vi "Controller Data Server Loop.vi"(4 "Log File Reference":refnum<file>, 7 "Sync Objects":T1, 8 "error in (no error)":errorcluster, 11 "FOFB Configuration":T5={"FOFB Parameters"={"Network"={"FOFB Controller IP"="", "LNLS Control Network IP"="", "LNLS Control Network Power Supplies TCP Port"=0, "LNLS Control Network FOFB Configuration TCP Port"=0, "Data Server TCP Port"=0, "Monitoring Data TCP Port"=0, "Configuration GUI TCP Port"=0, "TCP Listening Timeout"=0}, "Fast Acquisition"={"Acquisition Period"=0, "Data Buffer Size"=0, "Monitoring Period"=0}, "Response Matrix Measurement"={"Step Amplitude"=0.0, "Time Between Steps"=0, "Step Duration"=0, "Number of Averages"=0}, "Correction Algorithm"={"Correction Period"=0, "Reference Orbit Path"=path "", "Response Matrix Path"=path "", "Correction Matrix Path"=path "", "Horizontal Correction Factor"=0.0, "Vertical Correction Factor"=0.0, "Beam Current FOFB Threshold"=0.0, "Decouple H-V"=FALSE, "Use Additional BPM LPF"=FALSE, "BPM LPF Cutoff"=0.0}, "Acquisition Network"=[], "Actuation Network"=[]}, "Number of Acquisition Chassis"=0, "Number of Actuation Chassis"=0, "Number of BPM Readings"=0, "BPM Reading Names"=[], "Selected BPM Readings"=[0, 1, 2, 3, 4, 5, 6, 7, 8, 9, 10, 11, 12, 13, 14, 15, 16, 17, 18, 19, 20, 21, 22, 23, 24, 25, 26, 27, 28, 29, 30, 31, 32, 33, 34, 35, 36, 37, 38, 39, 40, 41, 42, 43, 44, 45, 46, 47, 48, 49], "Number of Correctors"=0, "Corrector Names"=[], "Selected Correctors"=[0, 1, 2, 3, 4, 5, 6, 7, 8, 9, 10, 11, 12, 13, 14, 15, 16, 17, 18, 19, 20, 21, 22, 23, 24, 25, 26, 27, 28, 29, 30, 31, 32, 33, 34, 35, 36, 37, 38, 39, 40, 41, 42, 43, 44, 45, 46, 47, 48, 49], "Reference Orbit"=[], "Response Matrix"=[], "Correction Matrix"=[], "Acquisition Chassis Names"=[], "Actuation Chassis Names"=[], "Acquisition Variables"=[], "Actuation Variables"=[], "PS Matrix Mapping"=[], "Inverse PS Matrix Mapping"=[], "Response Matrix Beam Energy (MeV)"=0.0, "PID Parameters"=[], "BPM Planes"=[], "Corrector Planes"=[], "RMM Step Factor"=[]}) -> (0 "error out":errorcluster)   [LabVIEW 2011, in "Controller VIs.lvlib"]
uses:
  Controller VIs.lvlib
  Types Definitions/Type FOFB Configuration.ctl
  Types Definitions/Type FOFB Parameters.ctl
  Types Definitions/Type Network Configuration.ctl
  Types Definitions/Type FA Configuration.ctl
  Types Definitions/Type Response Matrix Measurement Configuration.ctl
  Types Definitions/Type Correction Algorithm Configuration.ctl
  Types Definitions/Type Acquisition Network Configuration.ctl
  Types Definitions/Type Actuation Network Configuration.ctl
  Types Definitions/Type PID Parameters.ctl
  Types Definitions/Type Synchronization Objects.ctl
  Types Definitions/Type Blocking Synchronization Objects.ctl
  Types Definitions/Type FA Request Parameters.ctl
  Types Definitions/Type BPM and PS select cluster.ctl
  Types Definitions/Type FA File Parameters.ctl
  Types Definitions/Type Monitoring Data.ctl
  Types Definitions/Type Diagnostics Data.ctl
  Types Definitions/Type CPU Loads Array.ctl
  Types Definitions/Type CPU Loads.ctl
  Types Definitions/Type Non-blocking Synchronization Objects.ctl
  Types Definitions/Type FOFB Variables.ctl
  Types Definitions/Type Actuation State.ctl
  Types Definitions/Type TCP State.ctl
  <vilib>/Platform/TimedLoop/XDataNode/timing_clust.ctl
  <vilib>/Platform/TimedLoop/XDataNode/nitl_modes.ctl
  <vilib>/Platform/TimedLoop/XDataNode/wakeup.ctl
  <vilib>/rtutility.llb/RT Debug String.vi
  <vilib>/Platform/TimedLoop/XDataNode/XDataNode.xnode
  Data Server VIs.lvlib
  Log VIs.lvlib
  Type Definitions.lvlib
  <vilib>/Platform/TimedLoop/XDataNode/XDNodeRunTimeDep.lvlib
  XML VIs.lvlib
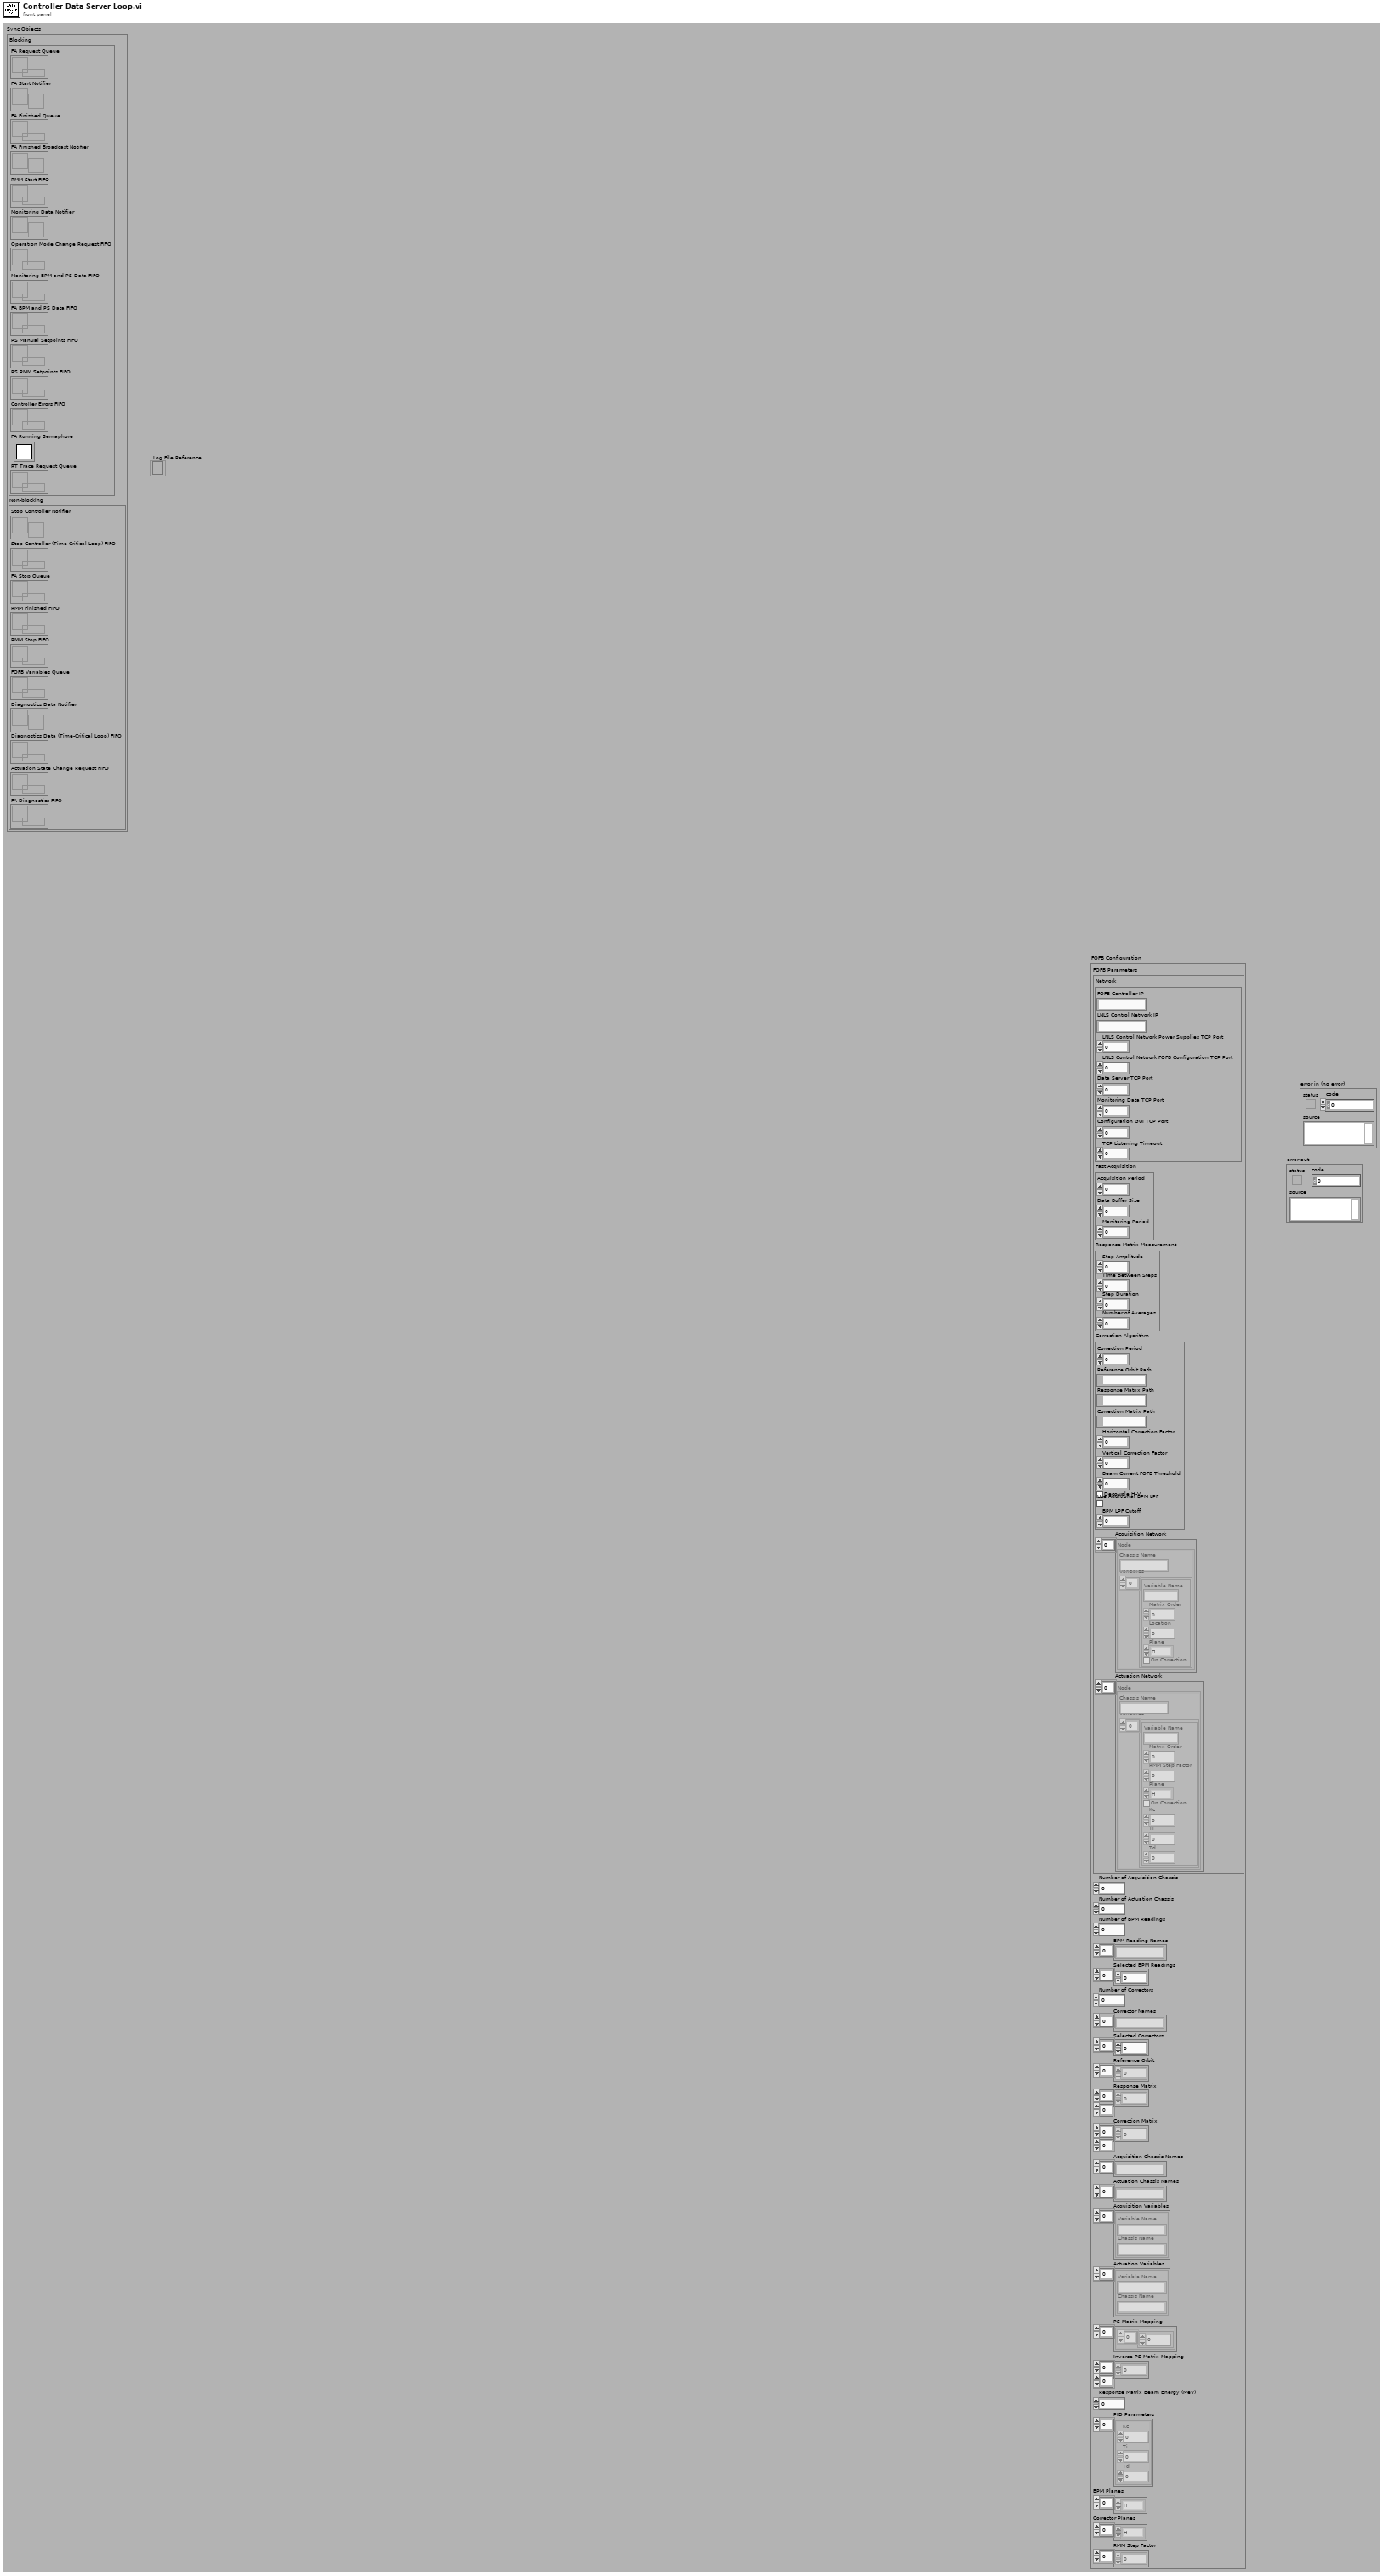
[diagram p1: front panel]
types:
  T1 = typedef "Type Definitions.lvlib/Type Synchronization Objects.ctl" = cluster{"Blocking":T2, "Non-blocking":T4}
  T2 = typedef "Type Definitions.lvlib/Type Blocking Synchronization Objects.ctl" = cluster{"FA Request Queue":refnum<queue>, "FA Start Notifier":refnum<notifier>, "FA Finished Queue":refnum<queue>, "FA Finished Broadcast Notifier":refnum<notifier>, "RMM Start FIFO":refnum<k33>, "Monitoring Data Notifier":refnum<notifier>, "Operation Mode Change Request FIFO":refnum<k33>, "Monitoring BPM and PS Data FIFO":refnum<k33>, "FA BPM and PS Data FIFO":refnum<k33>, "PS Manual Setpoints FIFO":refnum<k33>, "PS RMM Setpoints FIFO":refnum<k33>, "Controller Errors FIFO":refnum<k33>, "FA Running Semaphore":T3, "RT Trace Request Queue":refnum<queue>}
  T3 = typedef "Semaphore RefNum" = refnum<k1>
  T4 = typedef "Type Definitions.lvlib/Type Non-blocking Synchronization Objects.ctl" = cluster{"Stop Controller Notifier":refnum<notifier>, "Stop Controller (Time-Critical Loop) FIFO":refnum<k33>, "FA Stop Queue":refnum<queue>, "RMM Finished FIFO":refnum<k33>, "RMM Stop FIFO":refnum<k33>, "FOFB Variables Queue":refnum<queue>, "Diagnostics Data Notifier":refnum<notifier>, "Diagnostics Data (Time-Critical Loop) FIFO":refnum<k33>, "Actuation State Change Request FIFO":refnum<k33>, "FA Diagnostics FIFO":refnum<k33>}
  T5 = typedef "Type Definitions.lvlib/Type FOFB Configuration.ctl" = cluster{"FOFB Parameters":T6, "Number of Acquisition Chassis":i32, "Number of Actuation Chassis":i32, "Number of BPM Readings":i32, "BPM Reading Names":string[], "Selected BPM Readings":u32[], "Number of Correctors":i32, "Corrector Names":string[], "Selected Correctors":u32[], "Reference Orbit":dbl[], "Response Matrix":dbl[][], "Correction Matrix":dbl[][], "Acquisition Chassis Names":string[], "Actuation Chassis Names":string[], "Acquisition Variables":cluster{"Variable Name":string, "Chassis Name":string}[], "Actuation Variables":cluster{"Variable Name":string, "Chassis Name":string}[], "PS Matrix Mapping":cluster{u32[]}[], "Inverse PS Matrix Mapping":u32[][], "Response Matrix Beam Energy (MeV)":dbl, "PID Parameters":T13[], "BPM Planes":enum8{"H", "V"}[], "Corrector Planes":enum8{"H", "V"}[], "RMM Step Factor":dbl[]}
  T6 = typedef "Type Definitions.lvlib/Type FOFB Parameters.ctl" = cluster{"Network":T7, "Fast Acquisition":T8, "Response Matrix Measurement":T9, "Correction Algorithm":T10, "Acquisition Network":T11, "Actuation Network":T12}
  T7 = typedef "Type Definitions.lvlib/Type Network Configuration.ctl" = cluster{"FOFB Controller IP":string, "LNLS Control Network IP":string, "LNLS Control Network Power Supplies TCP Port":u16, "LNLS Control Network FOFB Configuration TCP Port":u16, "Data Server TCP Port":u16, "Monitoring Data TCP Port":u16, "Configuration GUI TCP Port":u16, "TCP Listening Timeout":i32}
  T8 = typedef "Type Definitions.lvlib/Type FA Configuration.ctl" = cluster{"Acquisition Period":u32, "Data Buffer Size":u32, "Monitoring Period":u32}
  T9 = typedef "Type Definitions.lvlib/Type Response Matrix Measurement Configuration.ctl" = cluster{"Step Amplitude":dbl, "Time Between Steps":u32, "Step Duration":u32, "Number of Averages":u32}
  T10 = typedef "Type Definitions.lvlib/Type Correction Algorithm Configuration.ctl" = cluster{"Correction Period":u32, "Reference Orbit Path":path, "Response Matrix Path":path, "Correction Matrix Path":path, "Horizontal Correction Factor":dbl, "Vertical Correction Factor":dbl, "Beam Current FOFB Threshold":dbl, "Decouple H-V":bool, "Use Additional BPM LPF":bool, "BPM LPF Cutoff":dbl}
  T11 = typedef "Type Definitions.lvlib/Type Acquisition Network Configuration.ctl" = cluster{"Chassis Name":string, "Variables":cluster{"Variable Name":string, "Matrix Order":u32, "Location":dbl, "Plane":enum8{"H", "V"}, "On Correction":bool}[]}[]
  T12 = typedef "Type Definitions.lvlib/Type Actuation Network Configuration.ctl" = cluster{"Chassis Name":string, "Variables":cluster{"Variable Name":string, "Matrix Order":u32, "RMM Step Factor":dbl, "Plane":enum8{"H", "V"}, "On Correction":bool, "Kc":dbl, "Ti":dbl, "Td":dbl}[]}[]
  T13 = typedef "Type Definitions.lvlib/Type PID Parameters.ctl" = cluster{"Kc":fxp<+/-,16,8>, "Ti":fxp<+/-,16,8>, "Td":fxp<+/-,16,8>}
  T14 = typedef "Type Definitions.lvlib/Type TCP State.ctl" = enum16{"Idle", "Wait Connection", "Read Data", "Process Data", "Write Data", "Close Connection"}
  T15 = typedef "XDNodeRunTimeDep.lvlib/timing_clust.ctl" = cluster{"Expected End [f-1]":u64, "Actual End [f-1]":u64, "Finished Late? [f-1]":bool, "Expected End [i-1]":u64, "Actual End [i-1]":u64, "Finished Late? [i-1]":bool, "Expected Start [i]":u64, "Actual Start [i]":u64, "Expected Start [f]":u64, "Actual Start [f]":u64, "Source Name":string, "Structure Name":string, "Period":i64, "Deadline":i64, "Offset":i64, "Start":i64, "Priority":i32, "Timeout":i32, "Mode":T16, "Wakeup Reason":T17, "Error":errorcluster, "Source Type":string, "Secondary Source Type":string, "Global End Time":u64, "Global Start Time":u64, "Frame Duration":u64, "Iteration Duration":u64, "Assigned CPU":i32, "I/O Scan Engine Mode":u32}
  T16 = typedef "XDNodeRunTimeDep.lvlib/nitl_modes.ctl" = enum32{"No Change", "Process missed periods, maintain original phase", "Discard missed periods, maintain original phase", "Process missed periods, ignore original phase", "Discard missed periods, ignore original phase"}
  T17 = typedef "XDNodeRunTimeDep.lvlib/wakeup.ctl" = enum32{"Normal", "Aborted", "Asynchronous wakeup", "Timing source error", "Timed loop error", "Timeout"}
  T18 = enum16{"Standard", "Buffered", "CRLF", "Immediate"}
  T19 = typedef "Type Definitions.lvlib/Type FA Request Parameters.ctl" = cluster{"Number of Samples":u32, "BPM and PS Selection":T20, "Filename":string}
  T20 = typedef "Type Definitions.lvlib/Type BPM and PS select cluster.ctl" = cluster{"BPM index array":u32[], "PS index array ":u32[]}
  T21 = typedef "Type Definitions.lvlib/Type Data Server Command ID.ctl" = enum16{"None", "FA_Start", "FA_Stop", "Update_Controller"}
  T22 = typedef "Type Definitions.lvlib/Type FOFB Variables.ctl" = cluster{"Correction Period":u32, "Reference Orbit":dbl[], "Response Matrix":dbl[][], "Correction Matrix":dbl[][], "Decouple H-V":bool, "Horizontal Correction Factor":dbl, "Vertical Correction Factor":dbl, "Selected BPM Readings":u32[], "Selected Correctors":u32[], "BPM Planes":enum8{"H", "V"}[], "Corrector Planes":enum8{"H", "V"}[], "Beam Current FOFB Threshold":dbl, "Response Matrix Beam Energy (MeV)":dbl}
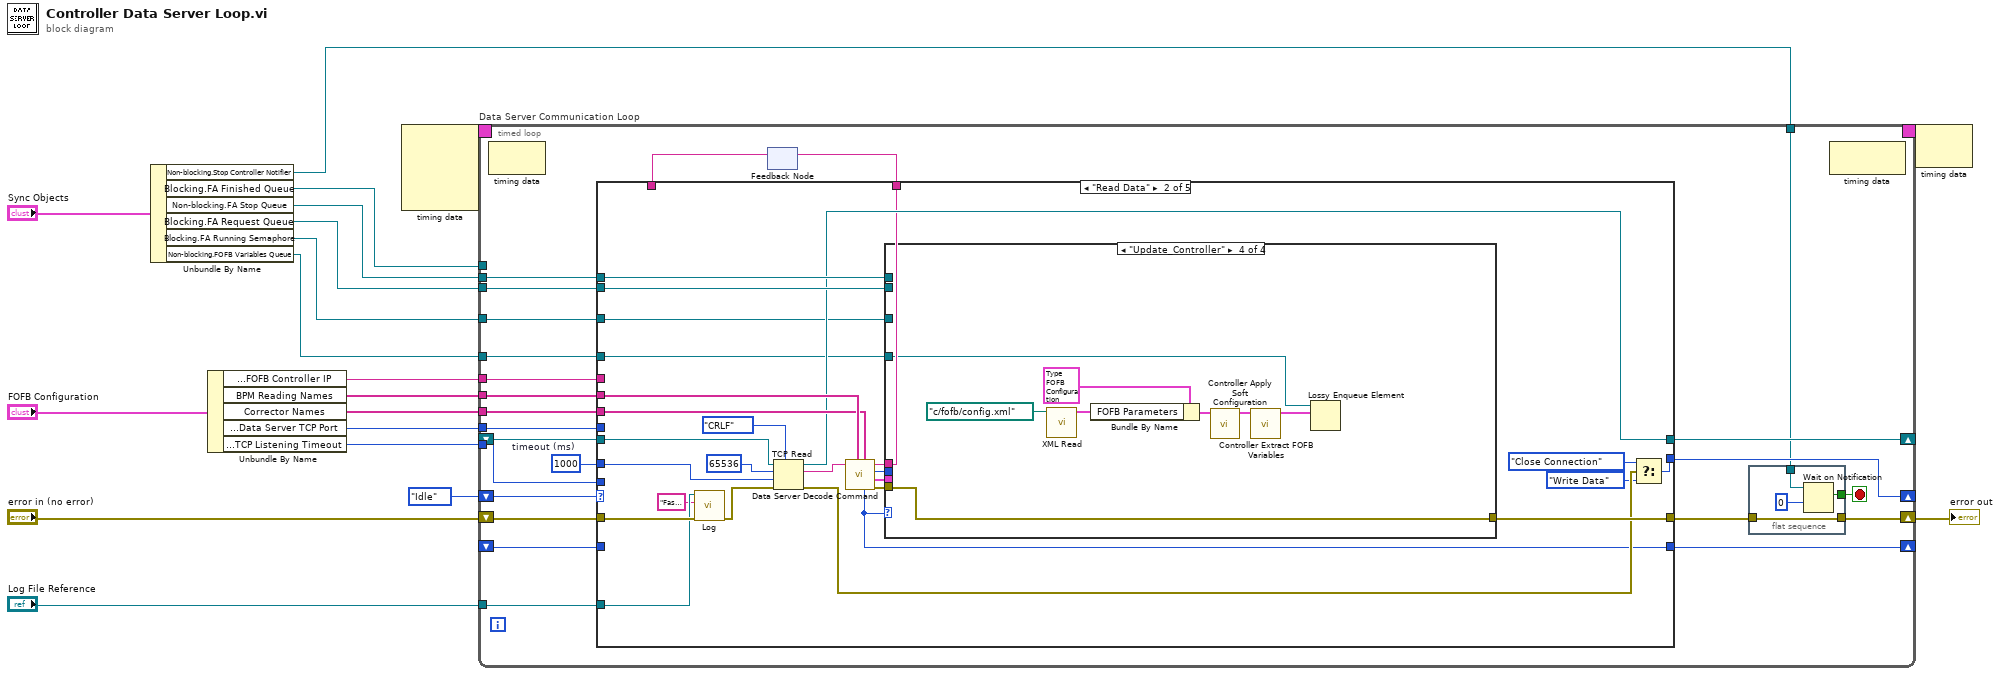
[diagram p0: block diagram]
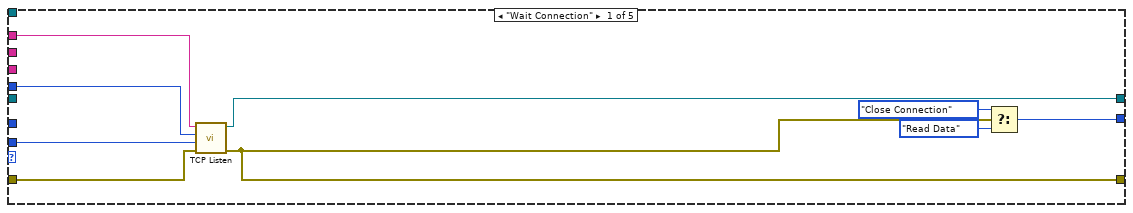
[diagram p2: hidden frame]
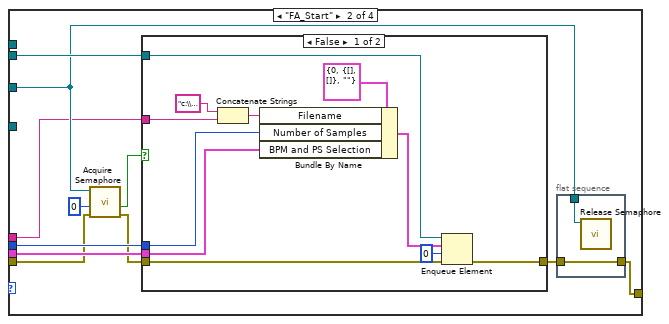
[diagram p4: hidden frame]
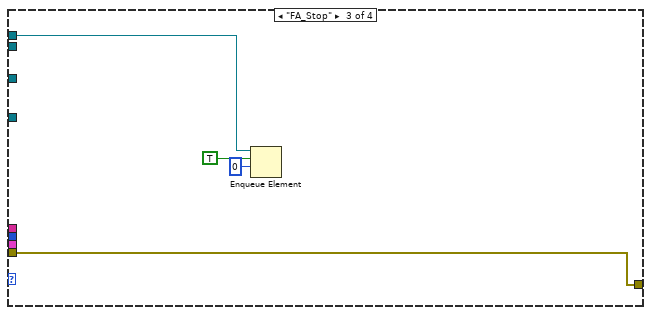
[diagram p6: hidden frame]
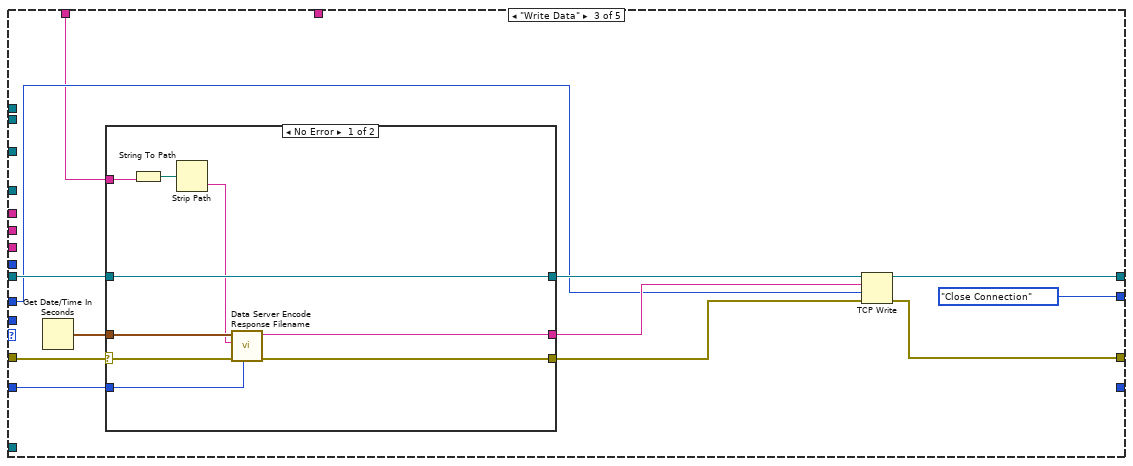
[diagram p7: hidden frame]
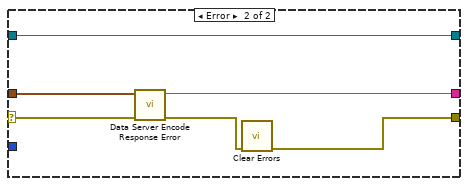
[diagram p8: hidden frame]
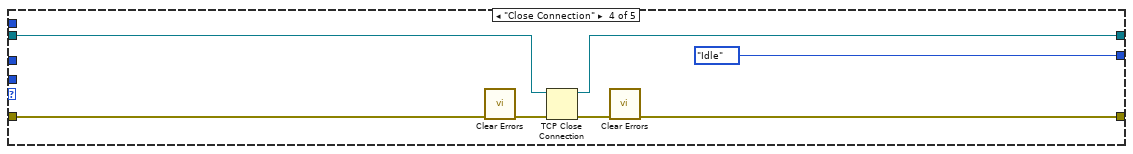
[diagram p9: hidden frame]
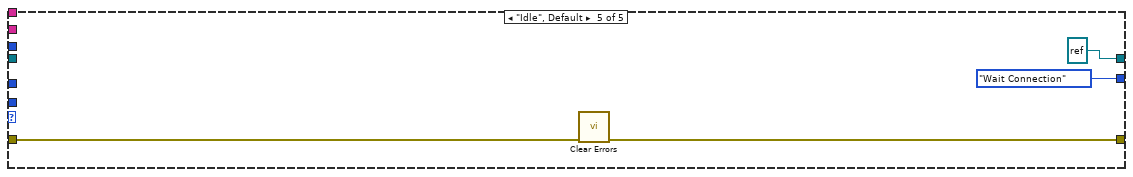
[diagram p10: hidden frame]
diagram:
  n1 = Unbundle By Name("Sync Objects") -> ("Non-blocking.Stop Controller Notifier"=w9:refnum<notifier>, "Blocking.FA Finished Queue"=w5:refnum<queue>, "Non-blocking.FA Stop Queue"=w7:refnum<queue>, "Blocking.FA Request Queue"=w8:refnum<queue>, "Blocking.FA Running Semaphore"=w4:T3, "Non-blocking.FOFB Variables Queue"=w1:refnum<queue>)
  n2 = Unbundle By Name("FOFB Configuration") -> ("FOFB Parameters.Network.FOFB Controller IP"=w12:string, "BPM Reading Names"=w13:string[], "Corrector Names"=w14:string[], "FOFB Parameters.Network.Data Server TCP Port"=w10:u16, "FOFB Parameters.Network.TCP Listening Timeout"=w6:i32)
  n3 = node-c288() -> (w3:T15)  [unwired: 4 in]
  n4 = timed-loop "Data Server Communication Loop" {
    shift-right: [w42] -> _
    shift-left: _ -> [w39]
    shift-right: [w41] -> _
    shift-left: Type_TCP_State."Idle" ("f") -> [w43]
    shift-right: [w29] -> w16
    shift-left: "error in (no error)" -> [w40]
    tunnel: w13 -> [w37]
    tunnel: w14 -> [w36]
    tunnel: w12 -> [w35]
    tunnel: w10 -> [w33]
    tunnel: w9 -> [w32]
    tunnel: "Log File Reference" -> [w31]
    tunnel: w8 -> [w28]
    tunnel: w7 -> [w27]
    tunnel: w6 -> [w26]
    shift-right: [w25] -> _
    shift-left: _ -> [w24]
    tunnel: w5 -> [_]
    tunnel: w4 -> [w23]
    timing: w3 -> [_]
    timing-out: [_] -> w2
    tunnel: w1 -> [w20]
    stop <- w34 stop-if-true
    w38 = 1000  # timeout (ms)
    # "ms"
    n5 = node-c288() -> ()  [unwired: 1 in, 1 out]
    n6 = feedback #1() -> (w22:string)  [unwired: 1 in]
    n7 = case shown="\"Read Data\"" w43 {
      tunnel: [w58 w62 w129 w154 refnum<k5> refnum ("connection ID")] -> w42
      tunnel: [w55 w68 Type_TCP_State."Close Connection" ("f") Type_TCP_State."Idle" ("f") Type_TCP_State."Wait Connection" ("f")] -> w41
      tunnel: [w50 w69 w125 w153 w157] -> w30
      tunnel: w40 -> [w51 w77 w134 w150 w158]
      tunnel: w39 -> [_ w82 w132 w155 _]
      tunnel: w38 -> [_ w81 w127 _ _]
      tunnel: w37 -> [_ w79 _ _ _]
      tunnel: w36 -> [_ w78 _ _ _]
      tunnel: w35 -> [w54 _ _ _ _]
      tunnel: w33 -> [w53 _ _ _ _]
      tunnel: w31 -> [_ w75 _ _ _]
      tunnel: w28 -> [_ w73 _ _ _]
      tunnel: w27 -> [_ w64 _ _ _]
      tunnel: w26 -> [w52 _ _ _ _]
      tunnel: w24 -> [_ _ w124 _ _]
      tunnel: [_ w63 _ _ _] -> w25
      tunnel: w23 -> [_ w61 _ _ _]
      tunnel: w22 -> [_ _ w123 _ _]
      tunnel: [_ w60 _ _ _] -> w21
      tunnel: w20 -> [_ w59 _ _ _]
      frame "Wait Connection" {
        n8 = call <vilib>:"TCP Listen.vi"("error in (no error)"=w51, "timeout ms (wait forever: -1)"=w52, "port"=w53, "service name"=w54) -> ("error out"=w50:errorcluster, "connection ID"=w58:refnum<k5>)  [unwired: 3 in, 3 out]
        n9 = Select(t=Type_TCP_State."Close Connection" ("f"), s=w50, f=Type_TCP_State."Read Data") -> (s? t:f=w55:T14)
      }
      frame "Read Data" {
        n10 = call "Log.vi"("error in (no error)"=w77, "String"="Fast Acquisition requested by user.", "Log File Reference"=w75) -> ("error out"=w76:errorcluster)  [unwired: 7 in, 1 out]
        n11 = TCP Read(connection ID=w82, bytes to read=65536, error in (no error)=w76, 7:T18."CRLF" ("mode (standard)"), 9:w81) -> (connection ID out=w62:refnum<k5>, data out=w80:string, error out=w66:errorcluster)
        n12 = call "Data Server Decode Command.vi"("Corrector names"=w78, "BPM names"=w79, "Input string"=w80) -> ("error out"=w70:errorcluster, "BPM and PS index"=w71:T20, "Number of samples"=w72:u32, "Filename"=w60:string, "Command ID"=w63:T21)  [unwired: 4 in]
        n13 = case shown="\"Update_Controller\"" w63 {
          tunnel: w73 -> [_ w96 _ _]
          tunnel: w72 -> [_ w95 _ _]
          tunnel: w71 -> [_ w94 _ _]
          tunnel: w70 -> [w85 w92 w114 w122]
          tunnel: [w85 w87 w114 w122] -> w69
          tunnel: w64 -> [_ _ w113 _]
          tunnel: w61 -> [_ w89 _ _]
          tunnel: w60 -> [_ w86 _ _]
          tunnel: w59 -> [_ _ _ w116]
          frame "None", Default {
          }
          frame "FA_Start" {
            n14 = call <vilib>:"Acquire Semaphore.vi"("error in (no error)"=w92, "ms timeout (-1)"=0, "semaphore"=w89) -> ("error out"=w91:errorcluster, "timed out"=w90:bool)  [unwired: 2 in, 1 out]
            n15 = case shown="False" w90 {
              tunnel: w96 -> [w106 _]
              tunnel: w95 -> [w108 _]
              tunnel: w94 -> [w107 _]
              tunnel: w86 -> [w101 _]
              tunnel: [w102 w110] -> w88
              tunnel: w91 -> [w104 w110]
              frame False {
                n16 = Concatenate Strings("c:\\fofb\\FA Data\\" ("string"), w101) -> (w99:string)
                n17 = Bundle By Name(cluster=T19 {"Number of Samples"=0, "BPM and PS Selection"={"BPM index array"=[], "PS index array "=[]}, "Filename"=""} ("notification"), "Filename"=w99, "Number of Samples"=w108, "BPM and PS Selection"=w107) -> (w105:T19)
                n18 = Enqueue Element(queue=w106, element=w105, timeout in ms (-1)=0, error in (no error)=w104) -> (error out=w102:errorcluster)  [unwired: 2 out]
              }
              frame True {
              }
            }
            n19 = flat-sequence {
              tunnel: w89 -> [w98]
              tunnel: w88 -> [w97]
              tunnel: [w97] -> w87
              frame #0 {
                n20 = call <vilib>:"Release Semaphore.vi"("semaphore"=w98) -> ()  [unwired: 5 in, 2 out]
              }
            }
          }
          frame "FA_Stop" {
            n21 = Enqueue Element(queue=w113, element=TRUE ("notification"), timeout in ms (-1)=0) -> ()  [unwired: 1 in, 3 out]
          }
          frame "Update_Controller" {
            n22 = call "XML Read.vi"("XML File Path In"=path "c:/fofb/config.xml" ("Configuration File Path")) -> ("FOFB Parameters"=w120:T6)  [unwired: 9 in, 1 out]
            n23 = Bundle By Name(cluster=T5 {"FOFB Parameters"={"Network"={"FOFB Controller IP"="", "LNLS Control Network IP"="", "LNLS Control Network Power Supplies TCP Port"=0, "LNLS Control Network FOFB Configuration TCP Port"=0, "Data Server TCP Port"=0, "Monitoring Data TCP Port"=0, "Configuration GUI TCP Port"=0, "TCP Listening Timeout"=0}, "Fast Acquisition"={"Acquisition Period"=0, "Data Buffer Size"=0, "Monitoring Period"=0}, "Response Matrix Measurement"={"Step Amplitude"=0.0, "Time Between Steps"=0, "Step Duration"=0, "Number of Averages"=0}, "Correction Algorithm"={"Correction Period"=0, "Reference Orbit Path"=path "", "Response Matrix Path"=path "", "Correction Matrix Path"=path "", "Horizontal Correction Factor"=0.0, "Vertical Correction Factor"=0.0, "Beam Current FOFB Threshold"=0.0, "Decouple H-V"=FALSE, "Use Additional BPM LPF"=FALSE, "BPM LPF Cutoff"=0.0}, "Acquisition Network"=[], "Actuation Network"=[]}, "Number of Acquisition Chassis"=0, "Number of Actuation Chassis"=0, "Number of BPM Readings"=0, "BPM Reading Names"=[], "Selected BPM Readings"=[], "Number of Correctors"=0, "Corrector Names"=[], "Selected Correctors"=[], "Reference Orbit"=[], "Response Matrix"=[], "Correction Matrix"=[], "Acquisition Chassis Names"=[], "Actuation Chassis Names"=[], "Acquisition Variables"=[], "Actuation Variables"=[], "PS Matrix Mapping"=[], "Inverse PS Matrix Mapping"=[], "Response Matrix Beam Energy (MeV)"=0.0, "PID Parameters"=[], "BPM Planes"=[], "Corrector Planes"=[], "RMM Step Factor"=[]}, "FOFB Parameters"=w120) -> (w118:T5)
            n24 = call "Controller Apply Soft Configuration.vi"("FOFB Configuration"=w118) -> ("FOFB Configuration"=w117:T5)  [unwired: 9 in, 1 out]
            n25 = call "Controller Extract FOFB Variables.vi"("FOFB Configuration"=w117) -> ("FOFB Variables"=w115:T22)  [unwired: 9 in, 1 out]
            n26 = Lossy Enqueue Element(queue=w116, element=w115) -> ()  [unwired: 1 in, 4 out]
          }
        }
        n27 = Select(t=Type_TCP_State."Close Connection" ("f"), s=w66, f=Type_TCP_State."Write Data") -> (s? t:f=w68:T14)
      }
      frame "Write Data" {
        n28 = Get Date/Time In Seconds() -> (seconds since 1Jan1904=w133:timestamp)
        n29 = case shown="No Error" w134 {
          selector: w134 -> [w142 w149]
          tunnel: w133 -> [w143 w148]
          tunnel: [w139 w144] -> w130
          tunnel: w132 -> [w141 w147]
          tunnel: [w141 w147] -> w131
          tunnel: [w140 w145] -> w128
          tunnel: w123 -> [w138 _]
          tunnel: w124 -> [w135 _]
          frame No Error {
            n30 = String To Path(string=w138) -> (path=w137:path)
            n31 = Strip Path(path=w137) -> (name=w136:string)  [unwired: 1 out]
            n32 = call "Data Server Encode Response Filename.vi"("Command ID"=w135, "error in (no error)"=w142, "Filename"=w136, "Time Stamp"=w143) -> ("error out"=w140:errorcluster, "Output string"=w139:string)  [unwired: 6 in]
          }
          frame Error {
            n33 = call "Data Server Encode Response Error.vi"("error in (no error)"=w149, "Time Stamp"=w148) -> ("error out"=w146:errorcluster, "Output string"=w144:string)  [unwired: 8 in]
            n34 = call <vilib>:"Clear Errors.vi"("error in (no error)"=w146) -> ("error out"=w145:errorcluster)  [unwired: 6 in]
          }
        }
        n35 = TCP Write(connection ID=w131, data in=w130, error in (no error)=w128, 9:w127) -> (connection ID out=w129:refnum<k5>, error out=w125:errorcluster)  [unwired: 1 out]
      }
      frame "Close Connection" {
        n36 = call <vilib>:"Clear Errors.vi"("error in (no error)"=w150) -> ("error out"=w152:errorcluster)  [unwired: 6 in]
        n37 = TCP Close Connection(connection ID=w155, error in (no error)=w152) -> (connection ID out=w154:refnum<k5>, error out=w151:errorcluster)  [unwired: 1 in]
        n38 = call <vilib>:"Clear Errors.vi"("error in (no error)"=w151) -> ("error out"=w153:errorcluster)  [unwired: 6 in]
      }
      frame "Idle", Default {
        n39 = call <vilib>:"Clear Errors.vi"("error in (no error)"=w158) -> ("error out"=w157:errorcluster)  [unwired: 6 in]
      }
    }
    n40 = feedback-in #1(w21) -> ()
    n41 = flat-sequence {
      tunnel: [w48] -> w34
      tunnel: w32 -> [w47]
      tunnel: w30 -> [w46]
      tunnel: [w46] -> w29
      frame #0 {
        n42 = Wait on Notification(notifier=w47, timeout in ms (-1)=0) -> (notification=w48:bool)  [unwired: 2 in, 3 out]
      }
    }
    n43 = node-c288() -> ()  [unwired: 1 in, 1 out]
  }
  "error out" <- w16
  n44 = node-c288(w2) -> ()  [unwired: 1 out]
